vi "gfitsio-write-key-double.vi"(4 "units":string, 6 "comment":string, 7 "keyname":string, 8 "error in (no error)":errorcluster, 9 "value":dbl, 11 "gfits refnum":T1) -> (0 "error out":errorcluster, 3 "dup gfits refnum":T1)   [LabVIEW 2019, in "gfitsio.lvlib"]
doc: "Write a keyword of the appropriate data type into the current HDU. If the keyword already exists it will be overwritten. Otherwise a new keyword will be appended to the header."
uses:
  gfitsio.lvlib
  gfitsio-refnum.ctl
  cfitsio-datatypes.ctl
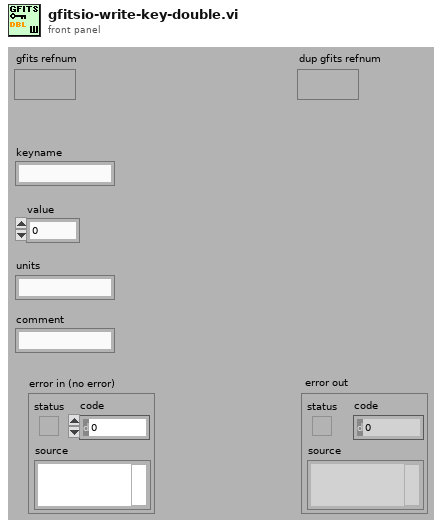
[diagram p1: front panel]
types:
  T1 = typedef "gfitsio.lvlib/gfitsio-refnum.ctl" = refnum<k1>
  T2 = typedef "gfitsio.lvlib/cfitsio-datatypes.ctl" = i32
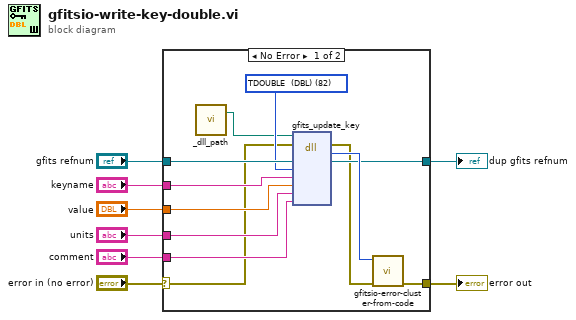
[diagram p0: block diagram]
diagram:
  n1 = case shown="No Error" "error in (no error)" {
    selector: "error in (no error)" -> [w11 w22]
    tunnel: [w19 w22] -> w4
    tunnel: "gfits refnum" -> [w17 w21]
    tunnel: [w18 w21] -> w7
    tunnel: "keyname" -> [w15 _]
    tunnel: "value" -> [w14 _]
    tunnel: "comment" -> [w13 _]
    tunnel: "units" -> [w12 _]
    frame No Error {
      w16 = T2 82 items=["TBIT"=1, "TBYTE  (U8)"=11, "TSBYTE  (I8)"=12, "TLOGICAL"=14, "TSTRING"=16, "TUSHORT  (U16)"=20, "TSHORT  (I16)"=21, "TUINT"=31, "TULONG  (U32)"=40, "TLONG  (I32)"=41, "TFLOAT  (SGL)"=42, "TLONGLONG  (I64)"=81, "TDOUBLE  (DBL)"=82, "TCOMPLEX  (CSG)"=83, "TDOUBLECOMPLEX  (CDB)"=163] ("cfitsio datatype")
      n2 = call "_dll_path.vi"() -> ("Path"=w9:path)  [unwired: 1 in]
      n3 = dll-call lib="?" fn="gfits_update_key"(path in=w9, error in=w11, "refnum"=w17, "datatype"=w16, "keyname"=w15, "value"=w14, "unit"=w12, "comment"=w13) -> (error out=w10:errorcluster, "return type"=w20:i32, "refnum"=w18:T1)  [unwired: 6 in, 1 out]
      n4 = call "gfitsio-error-cluster-from-code.vi"("error in (no error)"=w10, "error code"=w20) -> ("error out"=w19:errorcluster)  [unwired: 9 out]
    }
    frame Error {
    }
  }
  "error out" <- w4
  "dup gfits refnum" <- w7
